vi "2_4.vi"() -> ()   [LabVIEW 2017]
panel:
  out "A and B":bool
  out "A or B or C":bool
  out "not (A and C)":bool
  out "not B":bool
  out "A or B":bool
  in  "C":bool
  in  "B":bool
  in  "A":bool
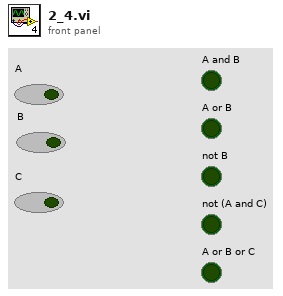
[diagram p1: front panel]
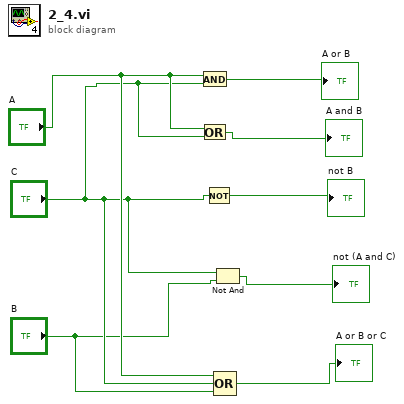
[diagram p0: block diagram]
diagram:
  n1 = And(x="A", y="C") -> (x .and. y?=→"A or B":bool)
  n2 = Or(x="A", y="C") -> (x .or. y?=→"A and B":bool)
  n3 = Not(x="C") -> (.not. x?=→"not B":bool)
  n4 = Not And(1:"B", 2:"C") -> (0:→"not (A and C)":bool)
  n5 = Compound Arithmetic op=OR("A", "C", "B") -> (→"A or B or C":bool)
